vi "Meas Proc QWTB Set Params Table.vi"(8 "error in":errorcluster, 10 "qwtb parameters":T1[](array[typedef]), 11 "param table ref":refnum<vi>) -> (0 "error out":errorcluster)   [LabVIEW 2020]
doc: "Takes previously parsed QWTB parameters and assigns them to the parameters table. Note the parameters order must match the algorithm parameters order."
uses:
  Meas Proc QWTB Algorithm Parameter Data.ctl
panel:
  out "data":string[][](array[string])
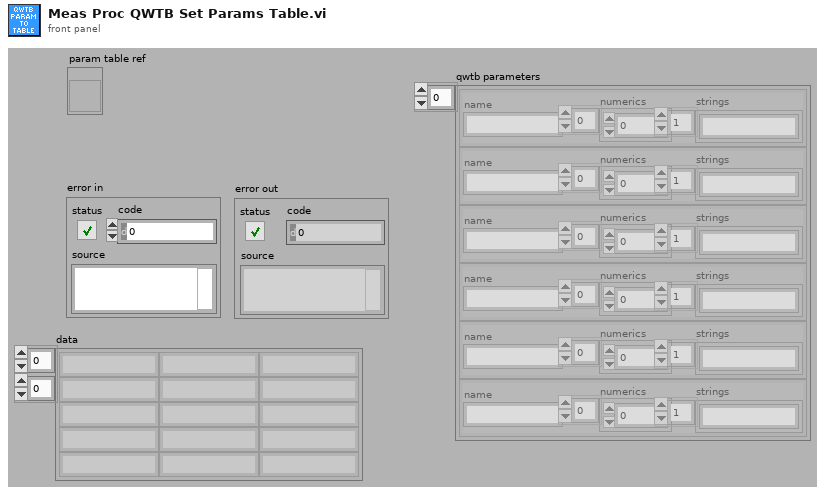
[diagram p1: front panel]
types:
  T1 = typedef "Meas Proc QWTB Algorithm Parameter Data.ctl" = cluster{"name":string, "numerics":dbl[], "strings":string[]}
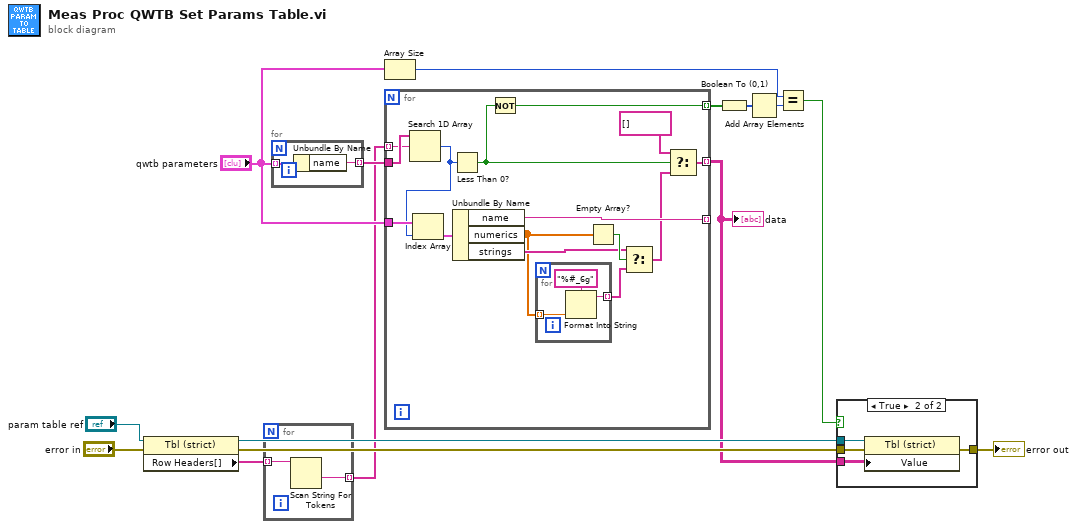
[diagram p0: block diagram]
diagram:
  n1 = property class="Tbl (strict)"(reference="param table ref", error in="error in") -> (reference out=w11:refnum<vi>, error out=w13:errorcluster, "Row Headers[]"=w2:string[])
  n2 = for {
    tunnel: w2 -> [w17] mode=indexing
    tunnel: [w16] -> w1 mode=indexing
    n3 = Scan String For Tokens(9:w17) -> (1:w16:string)  [unwired: 5 in, 3 out]
  }
  n4 = for {
    tunnel: "qwtb parameters" -> [w19] mode=indexing
    tunnel: [w18] -> w10 mode=indexing
    n5 = Unbundle By Name(w19) -> ("name"=w18:string)
  }
  n6 = Array Size(array="qwtb parameters") -> (size(s)=w4:i32)
  n7 = for {
    tunnel: "qwtb parameters" -> [w25]
    tunnel: [w30] -> _ mode=indexing
    tunnel: w1 -> [w21] mode=indexing
    tunnel: w10 -> [w22]
    tunnel: [w28] -> w8 mode=indexing
    tunnel: [w23] -> w9 mode=indexing
    n8 = Search 1D Array(1D array=w22, element=w21) -> (index of element=w20:i32)  [unwired: 1 in]
    n9 = Index Array(array=w25, index=w20) -> (element=w24:T1)
    n10 = Less Than 0?(x=w20) -> (x < 0?=w26:bool)
    n11 = Unbundle By Name(w24) -> ("name"=w30:string, "numerics"=w32:dbl[], "strings"=w33:string[])
    n12 = Not(x=w26) -> (.not. x?=w23:bool)
    n13 = for {
      tunnel: w32 -> [w37] mode=indexing
      tunnel: [w35] -> w31 mode=indexing
      n14 = Format Into String(format string="%#_6g", w37) -> (resulting string=w35:string)  [unwired: 2 in, 1 out]
    }
    n15 = Empty Array?(array=w32) -> (empty?=w34:bool)
    n16 = Select(t=w33, s=w34, f=w31) -> (s? t:f=w29:string[])
    n17 = Select(t=string[] [], s=w26, f=w29) -> (s? t:f=w28:string[])
  }
  "data" <- w8
  n18 = Boolean To (0,1)(Boolean=w9) -> (0, 1=w7:i16[])
  n19 = Add Array Elements(numeric array=w7) -> (sum=w5:i16)
  n20 = Equal?(x=w4, y=w5) -> (x = y?=w3:bool)
  n21 = case shown="True" w3 {
    tunnel: w13 -> [w38 w42]
    tunnel: w11 -> [_ w41]
    tunnel: [w38 w40] -> w15
    tunnel: w8 -> [_ w39]
    frame False {
    }
    frame True {
      n22 = property class="Tbl (strict)"(reference=w41, error in=w42, "Value"=w39) -> (error out=w40:errorcluster)  [unwired: 1 out]
    }
  }
  "error out" <- w15
